vi "Enter Row Cell Data.vi"(8 "error in (no error)":errorcluster, 9 "row index":i32, 10 "text":string, 11 "cell":refnum<k7>) -> (0 "error out":errorcluster)   [LabVIEW 2017, in "NI_ReportGenerationCore.lvlib"]
uses:
  <vilib>/Utility/NIReport.llb/NI_ReportGenerationCore.lvlib
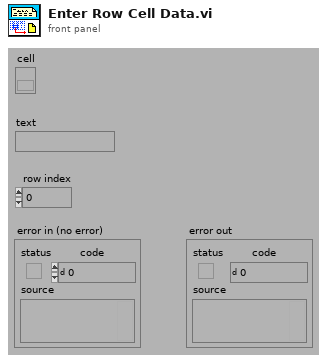
[diagram p1: front panel]
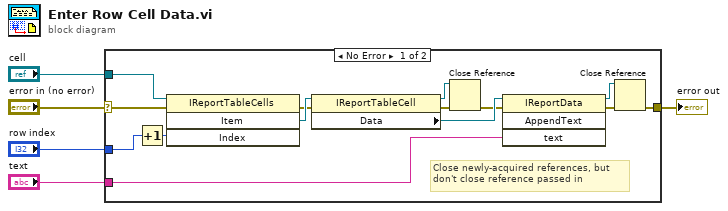
[diagram p0: block diagram]
diagram:
  n1 = case shown="No Error" "error in (no error)" {
    selector: "error in (no error)" -> [w12 w20]
    tunnel: "cell" -> [w17 _]
    tunnel: [w8 w20] -> w4
    tunnel: "text" -> [w16 _]
    tunnel: "row index" -> [w15 _]
    frame No Error {
      # "Close newly-acquired references, but\ndon't close reference passed in"
      n2 = Increment(x=w15) -> (x+1=w13:i32)
      n3 = invoke class="IReportTableCells" method="Item"(reference=w17, error in=w12, "Index"=w13) -> (error out=w14:errorcluster, "Item"=w18:refnum<k7>)  [unwired: 1 in, 2 out]
      n4 = property class="IReportTableCell"(reference=w18, error in=w14) -> (reference out=w10:refnum<k7>, error out=w11:errorcluster, "Data"=w19:refnum<k7>)
      n5 = Close Reference(reference=w10, error in (no error)=w11) -> (error out=w9:errorcluster)
      n6 = invoke class="IReportData" method="AppendText"(reference=w19, error in=w9, "text"=w16) -> (reference out=w6:refnum<k7>, error out=w7:errorcluster)  [unwired: 1 in, 2 out]
      n7 = Close Reference(reference=w6, error in (no error)=w7) -> (error out=w8:errorcluster)
    }
    frame Error {
    }
  }
  "error out" <- w4
